vi "z.stack.run_MD.vi"() -> ()   [LabVIEW 2012]
uses:
  Custom Controls/experiment type.ctl
  GFG/GFGnumericGet.vi
  GFG/GFGfpRefGet.vi
  GFG/GFGbooleanGet.vi
  GFG/GFG library.lvlib
panel:
  out "error out 2":errorcluster
  out "transposed array":dbl[][](array[numeric])
  out "data":dbl[][](array[numeric])
  in  "error in (no error)":errorcluster
  out "error out":errorcluster
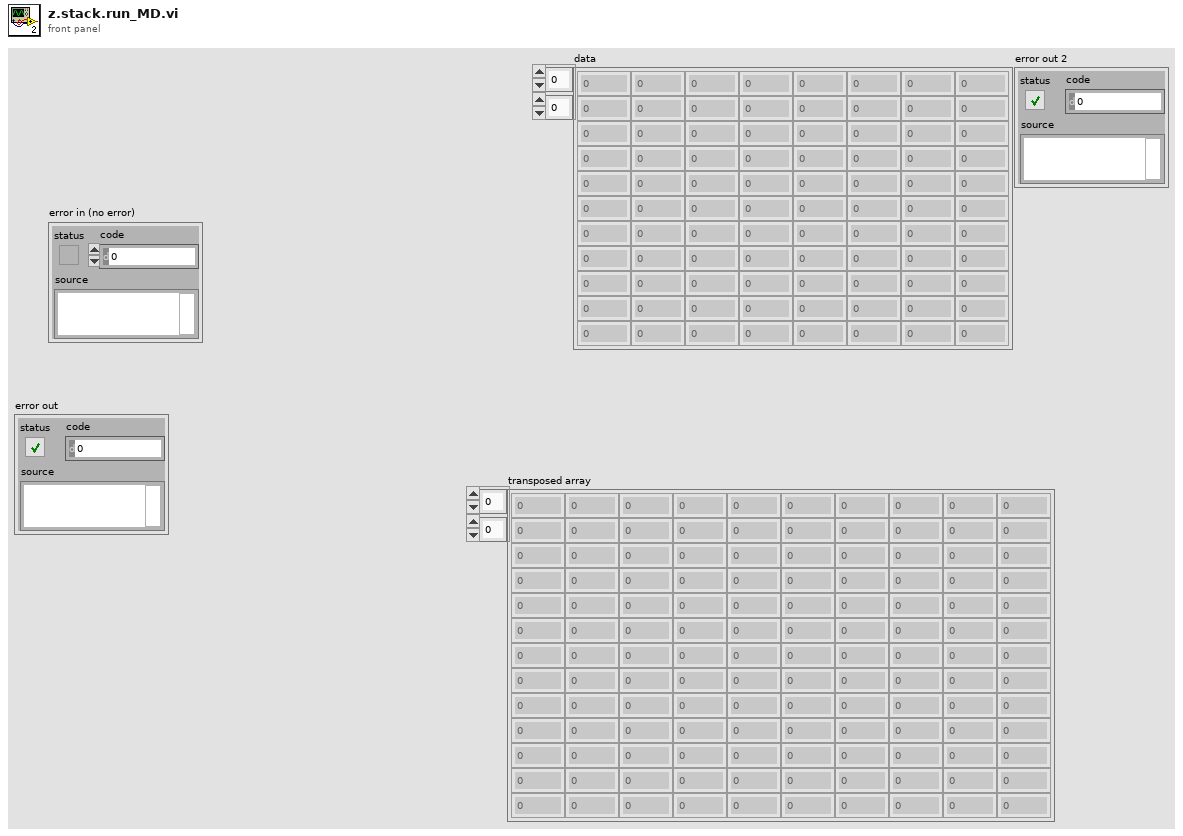
[diagram p1: front panel]
types:
  T1 = typedef "experiment type.ctl" = string
  T2 = enum8{"Enabled", "Disabled", "Disabled and Grayed Out"}
  T3 = cluster{"WaveformChartRef":refnum<vi>, "DigitalRef":refnum<vi>, "ArrayRef":refnum<vi>, "TabControlRef":refnum<vi>, "EnumRef":refnum<vi>, "RingRef":refnum<vi>, "BooleanRef":refnum<vi>, "KnobRef":refnum<vi>, "SlideRef":refnum<vi>, "PathRef":refnum<vi>, "StringRef":refnum<vi>, "ComboBox":refnum<vi>, "WaveformGraphRef":refnum<vi>}
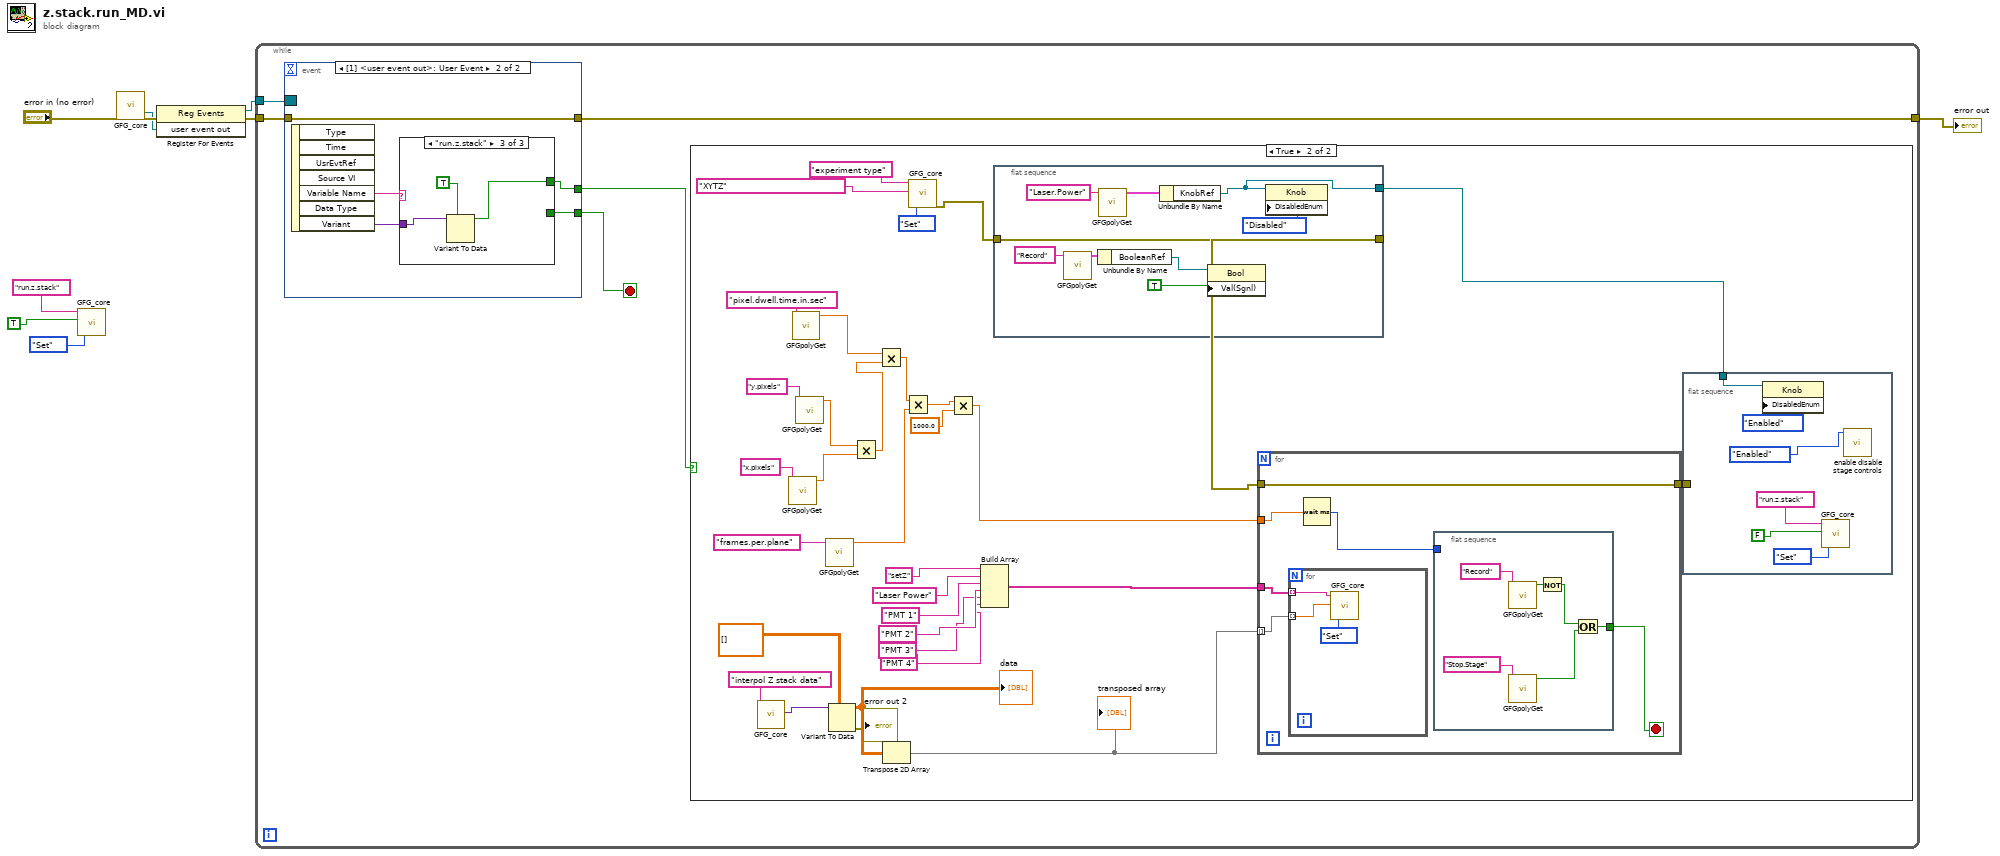
[diagram p0: block diagram]
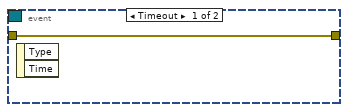
[diagram p3: hidden frame]
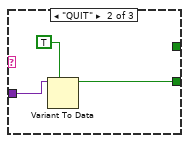
[diagram p5: hidden frame]
diagram:
  n1 = call "GFG_core.vi"("Variable Name in"="run.z.stack", "Variant in"=TRUE, "Action"=enum16{"Init", "Set", "Get"}."Set") -> ()  [unwired: 10 in, 7 out]
  n2 = call "GFG_core.vi"("error in (no error)"="error in (no error)") -> ("user event out"=w5:refnum<user-event>, "error out"=w6:errorcluster)  [unwired: 12 in, 5 out]
  n3 = register-events(error in=w6, w5) -> (reference out=w4:refnum<event-registration>, error out=w8:errorcluster)  [unwired: 1 in]
  n4 = while {
    tunnel: w4 -> [w14]
    tunnel: w8 -> [w13]
    tunnel: [w12] -> w9
    stop <- w11 stop-if-true
    n5 = event shown="[1] <user event out>: User Event" {
      selector: w14 -> [_ _]
      dyn-events: _ -> [_ _]
      timeout: _ -> [_ _]
      tunnel: w13 -> [w78 w83]
      tunnel: [w78 w83] -> w12
      tunnel: [_ w80] -> w11
      tunnel: [_ w79] -> w10
      event Timeout {
        n6 = event-data() -> ()  [unwired: 1 in, 2 out]
      }
      event User Event {
        n7 = event-data() -> ("Variable Name"=w82:string, "Variant"=w81:variant)  [unwired: 1 in, 5 out]
        n8 = case shown="\"run.z.stack\"" w82 {
          tunnel: w81 -> [_ w85 w88]
          tunnel: [_ w84 _] -> w80
          tunnel: [_ _ w87] -> w79
          frame "False", Default {
          }
          frame "QUIT" {
            n9 = Variant To Data(type=TRUE, Variant=w85) -> (data=w84:bool)  [unwired: 1 in, 1 out]
          }
          frame "run.z.stack" {
            n10 = Variant To Data(type=TRUE, Variant=w88) -> (data=w87:bool)  [unwired: 1 in, 1 out]
          }
        }
      }
    }
    n11 = case shown="True" w10 {
      frame False {
      }
      frame True {
        n12 = call "GFG_core.vi"("Variable Name in"="interpol Z stack data") -> ("Variant Out"=w33:variant)  [unwired: 12 in, 6 out]
        n13 = call-poly "GFGpolyGet.vi"("Variable Name in"="x.pixels") -> ("Numeric"=w43:dbl)  [unwired: 9 in, 1 out]
        n14 = call-poly "GFGpolyGet.vi"("Variable Name in"="pixel.dwell.time.in.sec") -> ("Numeric"=w42:dbl)  [unwired: 9 in, 1 out]
        n15 = call-poly "GFGpolyGet.vi"("Variable Name in"="y.pixels") -> ("Numeric"=w44:dbl)  [unwired: 9 in, 1 out]
        n16 = call-poly "GFGpolyGet.vi"("Variable Name in"="frames.per.plane") -> ("Numeric"=w38:dbl)  [unwired: 9 in, 1 out]
        n17 = Variant To Data(type=dbl[][] [] ("Interpolated Data"), Variant=w33) -> (data=w31:dbl[][], error out=→"error out 2":errorcluster)  [unwired: 1 in]
        "data" <- w31
        n18 = Multiply(x=w44, y=w43) -> (x*y=w41:dbl)
        n19 = Multiply(x=w42, y=w41) -> (x*y=w39:dbl)
        n20 = Transpose 2D Array(2D array=w31) -> (transposed array=w30:dbl[][])
        "transposed array" <- w30
        n21 = Multiply(x=w39, y=w38) -> (x*y=w37:dbl)
        n22 = call "GFG_core.vi"("Variable Name in"="experiment type", "Variant in"=T1 "XYTZ" ("experiment type"), "Action"=enum16{"Init", "Set", "Get"}."Set") -> ("error out"=w17:errorcluster)  [unwired: 10 in, 6 out]
        n23 = Multiply(x=w37, y=1000.0) -> (x*y=w35:dbl)
        n24 = Build Array("setZ" ("Variable Name in"), "Laser Power" ("Variable Name in"), "PMT 1" ("Variable Name in"), "PMT 2" ("Variable Name in"), "PMT 3" ("Variable Name in"), "PMT 4" ("Variable Name in")) -> (w23:string[])
        n25 = flat-sequence {
          tunnel: [w55] -> w18
          tunnel: w17 -> [w55]
          tunnel: [w48] -> w15
          frame #0 {
            n26 = call-poly "GFGpolyGet.vi"("Variable Name in"="Record") -> ("output cluster"=w54:T3)  [unwired: 9 in, 1 out]
            n27 = Unbundle By Name(w54) -> ("BooleanRef"=w53:refnum<vi>)
            n28 = call-poly "GFGpolyGet.vi"("Variable Name in"="Laser.Power") -> ("output cluster"=w50:T3)  [unwired: 9 in, 1 out]
            n29 = Unbundle By Name(w50) -> ("KnobRef"=w48:refnum<vi>)
            n30 = property class="Bool"(reference=w53, "Val(Sgnl)"=TRUE) -> ()  [unwired: 1 in, 2 out]
            n31 = property class="Knob"(reference=w48, "DisabledEnum"=T2."Disabled" ("Disabled")) -> ()  [unwired: 1 in, 2 out]
          }
        }
        n32 = for {
          tunnel: w35 -> [w68]
          tunnel: w30 -> [w67] mode=indexing
          tunnel: w23 -> [w66]
          tunnel: w18 -> [w63]
          tunnel: [w63] -> w19
          stop <- w64 stop-if-true
          n33 = for {
            tunnel: w67 -> [w76] mode=indexing
            tunnel: w66 -> [w77] mode=indexing
            n34 = call "GFG_core.vi"("Variable Name in"=w77, "Variant in"=w76, "Action"=enum16{"Init", "Set", "Get"}."Set") -> ()  [unwired: 10 in, 7 out]
          }
          n35 = Wait (ms)(milliseconds to wait=w68) -> (millisecond timer value=w65:u32)
          n36 = flat-sequence {
            tunnel: w65 -> [_]
            tunnel: [w70] -> w64
            frame #0 {
              n37 = call-poly "GFGpolyGet.vi"("Variable Name in"="Record") -> ("Boolean"=w72:bool)  [unwired: 10 in]
              n38 = call-poly "GFGpolyGet.vi"("Variable Name in"="Stop.Stage") -> ("Boolean"=w71:bool)  [unwired: 10 in]
              n39 = Not(x=w72) -> (.not. x?=w69:bool)
              n40 = Or(x=w69, y=w71) -> (x .or. y?=w70:bool)
            }
          }
        }
        n41 = flat-sequence {
          tunnel: w19 -> [_]
          tunnel: w15 -> [w57]
          frame #0 {
            n42 = property class="Knob"(reference=w57, "DisabledEnum"=T2."Enabled" ("Disabled")) -> ()  [unwired: 1 in, 2 out]
            n43 = call "GFG_core.vi"("Variable Name in"="run.z.stack", "Variant in"=FALSE, "Action"=enum16{"Init", "Set", "Get"}."Set") -> ()  [unwired: 10 in, 7 out]
            n44 = call "enable disable stage controls.vi"("Disabled"=T2."Enabled") -> ()  [unwired: 11 in]
          }
        }
      }
    }
  }
  "error out" <- w9
